vi "Configure.vi"(8 "error in (no error)":errorcluster, 11 "Behavior in":refnum<class "BehaviorData.lvclass">) -> (0 "error out":errorcluster, 3 "Behavior out":refnum<class "BehaviorData.lvclass">)   [LabVIEW 2010, in "BehaviorData.lvclass"]
uses:
  BehaviorData.lvclass
  Program Files/National Instruments/LabVIEW 2010/resource/objmgr/daqmx.rc
panel:
  in  "Recording Path":path
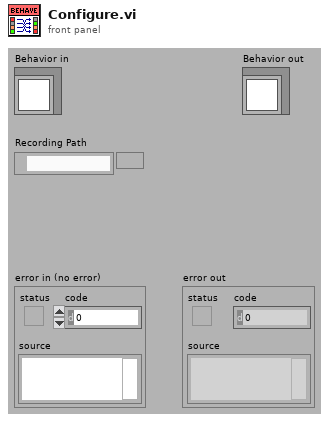
[diagram p1: front panel]
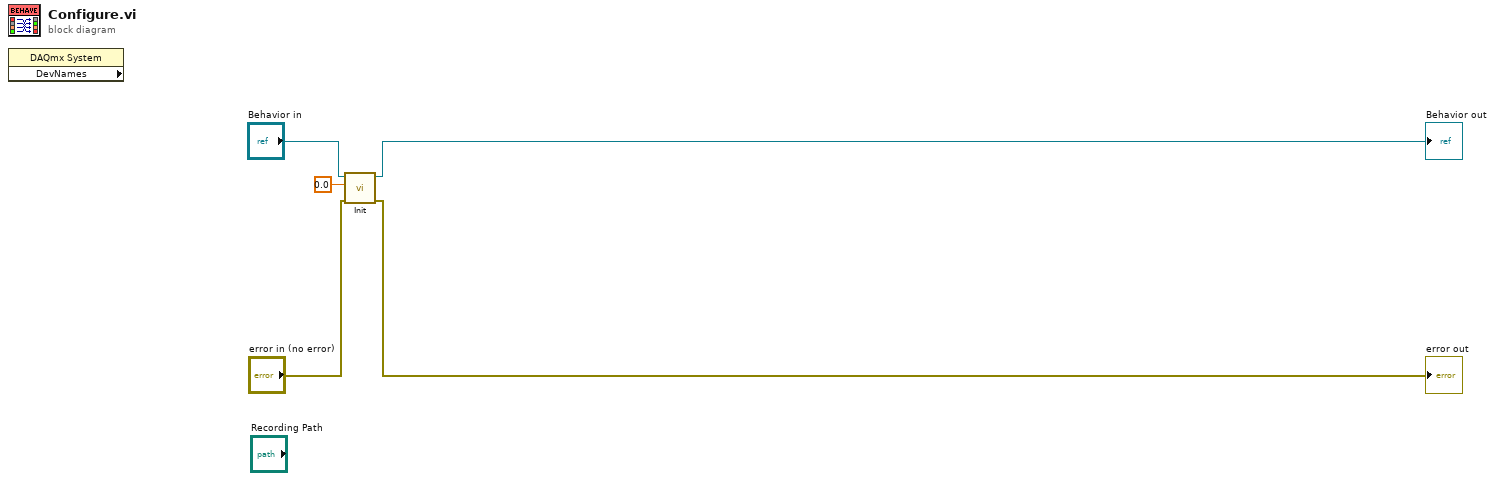
[diagram p0: block diagram]
diagram:
  n1 = property class="DAQmx System" props=["DevNames"]() -> ()  [unwired: 2 in, 3 out]
  n2 = call-dynamic "Init.vi"("error in (no error)"="error in (no error)", "Channel"=0.0, "AcquistionObject in"="Behavior in") -> ("error out"=→"error out":errorcluster, "AcquistionObject out"=→"Behavior out":refnum<class "BehaviorData.lvclass">)  [unwired: 7 in]
